vi "CreateCopyExactPackageWithReference.vi"(8 "Error In":errorcluster, 9 "Reference Package Version File (Optional)":path, 10 "Package Suffix":string="CE", 11 "Package Path":path) -> (0 "Error Out":errorcluster, 1 "Ignored Dependencies":string[](array[string]), 2 "Copy Exact Dependencies":string[](array[string]), 3 "Copy Exact Package Path":path)   [LabVIEW 2019, in "CEPM.lvlib"]
uses:
  CEPM.lvlib
  <vilib>/SLL Toolkit/SLL Table/_SubVIs/Get Table Data.vi
  <vilib>/SLL Toolkit/SLL File IO/Spreadsheet/SLL Spreadsheet.lvlib
  <vilib>/SLL Toolkit/SLL Table/SLL Table.lvclass
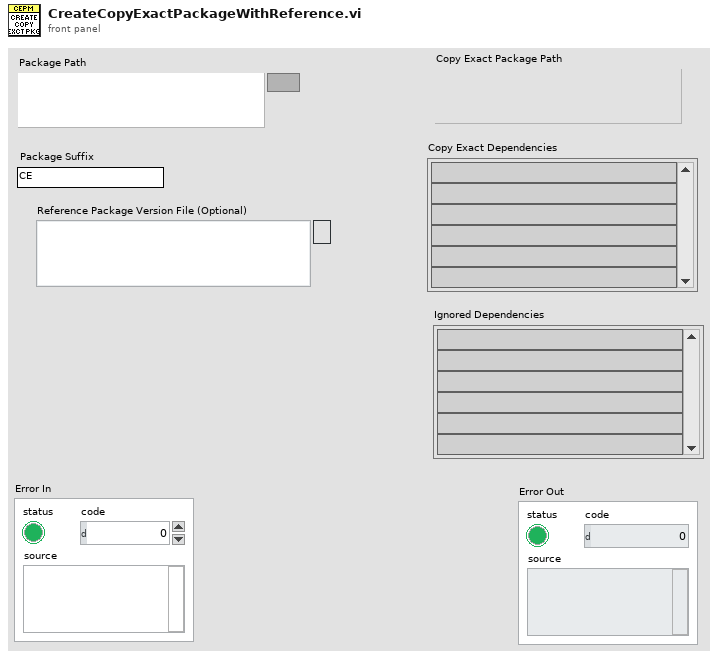
[diagram p1: front panel]
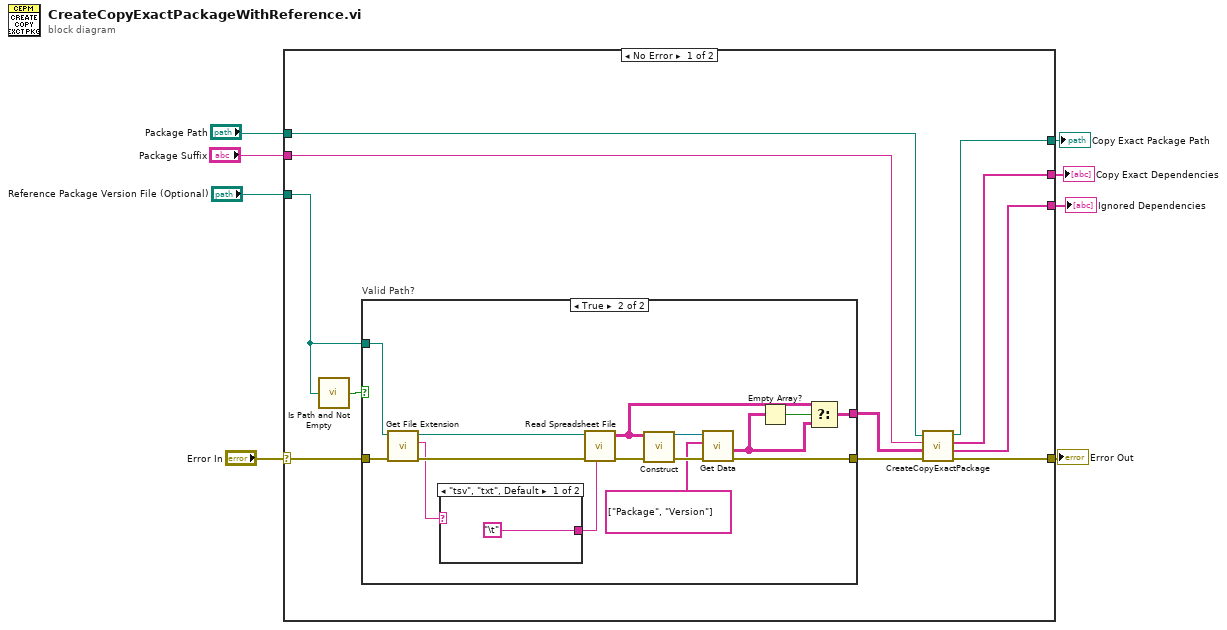
[diagram p0: block diagram]
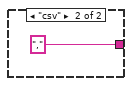
[diagram p3: hidden frame]
diagram:
  n1 = case shown="No Error" "Error In" {
    selector: "Error In" -> [w16 w38]
    tunnel: [w19 w38] -> w8
    tunnel: "Package Path" -> [w18 _]
    tunnel: "Package Suffix" -> [w17 _]
    tunnel: "Reference Package Version File (Optional)" -> [w14 _]
    tunnel: [w11 _] -> w3
    tunnel: [w10 _] -> w2
    tunnel: [w9 _] -> w1
    frame No Error {
      n2 = call <vilib>:"Is Path and Not Empty.vi"("path"=w14) -> ("Is Path and Not Empty?"=w13:bool)  [unwired: 4 in]
      n3 = case "Valid Path?" shown="True" w13 {
        tunnel: [w20 w28] -> w15
        tunnel: [_ w21] -> w12
        tunnel: w14 -> [_ w33]
        tunnel: w16 -> [w20 w35]
        frame False {
        }
        frame True {
          n4 = call <vilib>:"Get File Extension.vi"("error in (no error)"=w35, "file"=w33) -> ("error out"=w34:errorcluster, "lowercase file extension"=w31:string, "dup file"=w32:path)  [unwired: 5 in, 2 out]
          n5 = case shown="\"tsv\", \"txt\", Default" w31 {
            tunnel: ["\t" "," ("Delimiter (tab)")] -> w30
            frame "tsv", "txt", Default {
            }
            frame "csv" {
            }
          }
          n6 = call <vilib>:"Read Spreadsheet File.vi"("Delimiter (tab)"=w30, "error in (no error)"=w34, "File Path"=w32) -> ("error out"=w29:errorcluster, "2D Array"=w23:string[][])  [unwired: 7 in]
          n7 = call <vilib>:"Construct.vi"("error in (no error)"=w29, "2D String with Headers"=w23) -> ("error out"=w27:errorcluster, "Table"=w26:refnum<class "SLL Table.lvclass">)  [unwired: 8 in]
          n8 = call-poly <vilib>:"Get Data.vi"("error in (no error)"=w27, "Header Order[] (Optional)"=string[] ["Package", "Version"], "SLL Table in"=w26) -> ("error out"=w28:errorcluster, "2D Data Out[][]"=w22:string[][])  [unwired: 5 in, 2 out]
          n9 = Empty Array?(array=w22) -> (empty?=w24:bool)
          n10 = Select(t=w23, s=w24, f=w22) -> (s? t:f=w21:string[][])
        }
      }
      n11 = call "CreateCopyExactPackage.vi"("Error In"=w15, "Reference Package Versions (Optional)"=w12, "Package Suffix"=w17, "Package Path"=w18) -> ("Error Out"=w19:errorcluster, "Ignored Dependencies"=w9:string[], "Copy Exact Dependencies"=w10:string[], "Copy Exact Package Path"=w11:path)  [unwired: 4 in]
    }
    frame Error {
    }
  }
  "Error Out" <- w8
  "Copy Exact Package Path" <- w3
  "Copy Exact Dependencies" <- w2
  "Ignored Dependencies" <- w1
